vi "Set Channel.vi"(8 "error in (no error)":errorcluster, 10 "channelParameter":T1={"channel"=1, "gain"=1, "input"=enum."DIFF", "shunt"=1, "couple"=enum."DC", "filter"=enum."ON"} {"gain" items=["1x"=1, "10x"=10, "100x"=100, "1000x"=232]; "shunt" items=["Open"=0, "50 ohms"=50, "500 ohms"=500, "5k ohms"=5000, "50k ohms"=50000, "10M ohms"=10000000]; "channel" items=["1"=1, "2"=2, "3"=3, "4"=4, "5"=5, "6"=6, "7"=7, "8"=8]}, 11 "VISA Refnum in":refnum<visa-resource-name>="COM1") -> (0 "error out":errorcluster, 3 "VISA Refnum out":refnum<visa-resource-name>)   [LabVIEW 2019, in "KH7008.lvlib"]
uses:
  KH7008.lvlib
  typedefs/channelProperties--Cluster.ctl
  typedefs/channel--ring.ctl
  typedefs/gain--ring.ctl
  typedefs/input--Enum.ctl
  typedefs/shunt--ring.ctl
  typedefs/couple--Enum.ctl
  typedefs/filter--Enum.ctl
panel:
  out "Response":string
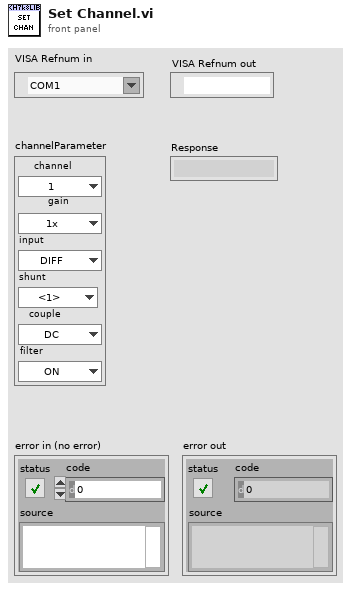
[diagram p1: front panel]
types:
  T1 = typedef "KH7008.lvlib/channelProperties--Cluster.ctl" = cluster{"channel":T2, "gain":T3, "input":T4, "shunt":T5, "couple":T6, "filter":T7}
  T2 = typedef "KH7008.lvlib/channel--ring.ctl" = u8
  T3 = typedef "KH7008.lvlib/gain--ring.ctl" = u8
  T4 = typedef "KH7008.lvlib/input--Enum.ctl" = enum8{"OFF", "SE+", "SE-", "DIFF"}
  T5 = typedef "KH7008.lvlib/shunt--ring.ctl" = u32
  T6 = typedef "KH7008.lvlib/couple--Enum.ctl" = enum8{"AC", "DC"}
  T7 = typedef "KH7008.lvlib/filter--Enum.ctl" = enum8{"OFF", "ON"}
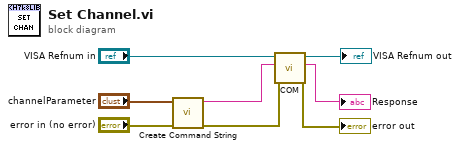
[diagram p0: block diagram]
diagram:
  n1 = call "Create Command String.vi"("error in (no error)"="error in (no error)", "Channel Params"="channelParameter") -> ("error out"=w4:errorcluster, "Command string"=w1:string)  [unwired: 8 in]
  n2 = call "COM.vi"("error in (no error)"=w4, "Command"=w1, "VISA Refnum in"="VISA Refnum in") -> ("error out"=→"error out":errorcluster, "Response"=→"Response":string, "VISA Refnum out"=→"VISA Refnum out":refnum<visa-resource-name>)  [unwired: 6 in]
